vi "Exit.vi"(8 "error in":errorcluster, 10 "Message Queues":T1, 11 "Notifiers":T2) -> (0 "error out":errorcluster)   [LabVIEW 2015, in "DAQ.lvlib"]
uses:
  DAQ.lvlib
  support/Notifiers/Notifiers.ctl
  support/Message Queue/All Message Queues.ctl
  support/Message Queue/Message Cluster.ctl
  support/Message Queue/Enqueue Message (Single).vi
  support/Message Queue/Message Queue.lvlib
  Support/Notifiers/Notifiers.lvlib
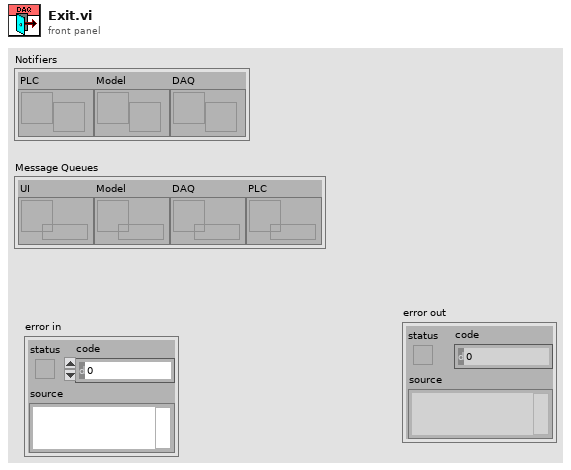
[diagram p1: front panel]
types:
  T1 = typedef "Message Queue.lvlib/All Message Queues.ctl" = cluster{"UI":refnum<queue>, "Model":refnum<queue>, "DAQ":refnum<queue>, "PLC":refnum<queue>}
  T2 = typedef "Notifiers.lvlib/Notifiers.ctl" = cluster{"PLC":refnum<notifier>, "Model":refnum<notifier>, "DAQ":refnum<notifier>}
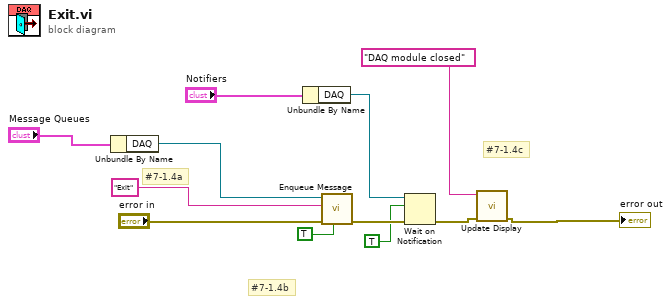
[diagram p0: block diagram]
diagram:
  # "#7-1.4c"
  # "#7-1.4b"
  # "#7-1.4a"
  n1 = Unbundle By Name("Message Queues") -> ("DAQ"=w7:refnum<queue>)
  n2 = Unbundle By Name("Notifiers") -> ("DAQ"=w8:refnum<notifier>)
  n3 = call-poly "Enqueue Message.vi"("Priority Message? (F)"=TRUE, "error in (no error)"="error in", "Message"="Exit", "Message Queue"=w7) -> ("error out"=w11:errorcluster)  [unwired: 6 in, 1 out]
  n4 = Wait on Notification(notifier=w8, ignore previous (F)=TRUE, error in (no error)=w11) -> (error out=w6:errorcluster)  [unwired: 1 in, 3 out]
  n5 = call "Update Display.vi"("error in"=w6, "Message string"="DAQ module closed") -> ("error out"=→"error out":errorcluster)  [unwired: 9 in]
